vi "GCFS.vi"() -> ()   [LabVIEW 2024]
uses:
  Ice-Nucleation-Controller/src/LabVIEW/DataCluster_GCFS.ctl
  <vilib>/userDefined/High Color/IMAQdx.ctl
  <vilib>/vision/Image Controls.llb/IMAQ Image.ctl
  <vilib>/Platform/TimedLoop/XDataNode/timing_clust.ctl
  <vilib>/Platform/TimedLoop/XDataNode/nitl_modes.ctl
  <vilib>/Platform/TimedLoop/XDataNode/wakeup.ctl
  <vilib>/vision/driver/IMAQdx.llb/IMAQdx Buffer Number Mode.ctl
  <vilib>/addons/_JKI Toolkits/State Machine/_JKI_lib_State_Machine.llb/Select State(s)_err__jki_lib_state_machine.vi
  <extravilib>/ChannelInstances/Stream-c(t'IMAQ Image.ctl',str)/Read With Abort.vi
  <extravilib>/ChannelInstances/Tag-t'DataCluster_GCFS.ctl'/Read With Abort.vi
  <extravilib>/ChannelInstances/Stream-c(t'IMAQ Image.ctl',str)/Write With Abort.vi
  <extravilib>/ChannelInstances/Tag-t'DataCluster_GCFS.ctl'/Write With Abort.vi
  <extravilib>/ChannelInstances/Stream-c(t'IMAQ Image.ctl',str)/EndpointRead.vi
  <extravilib>/ChannelInstances/Stream-c(t'IMAQ Image.ctl',str)/Endpoint.vi
  <extravilib>/ChannelInstances/Stream-c(t'IMAQ Image.ctl',str)/Instantiate.vi
  <extravilib>/ChannelInstances/Tag-t'DataCluster_GCFS.ctl'/Instantiate.vi
  <extravilib>/ChannelInstances/Stream-c(t'IMAQ Image.ctl',str)/)Channel.vi
  <resource>/ChannelSupport/_ChannelSupport/WaitIfNeeded.vi
  <extravilib>/ChannelInstances/Tag-t'DataCluster_GCFS.ctl'/EndpointRead.vi
  <vilib>/addons/_JKI Toolkits/State Machine/_JKI_lib_State_Machine.llb/Periodic Trigger__ogtk__JKI-SM__jki_lib_state_machine.vi
  <extravilib>/ChannelInstances/Tag-t'DataCluster_GCFS.ctl'/Endpoint.vi
  <vilib>/platform/TimedLoop/XDataNode/XDataNode.xnode
  <vilib>/vision/driver/NI_Vision_Acquisition_Software.lvlib
  <extravilib>/ChannelInstances/Tag-t'DataCluster_GCFS.ctl'.lvlib
  <vilib>/vision/NI_Vision_Development_Module.lvlib
  <vilib>/Platform/TimedLoop/XDataNode/XDNodeRunTimeDep.lvlib
  <extravilib>/ChannelInstances/Stream-c(t'IMAQ Image.ctl',str).lvlib
panel:
  in  "Get Image":bool
  out "Frezz Image":T1(plugin-control)
  out "Droplet binary":T1(plugin-control)
  out "Droplet Position":T1(plugin-control)
  out "Grap Image":T1(plugin-control)
  in  "Active":bool
  in  "Sample name":string
  in  "Grap Position Image":bool
  out "Statusstring":string
  out "Particle Measurements (Pixels) (Particle Analysis 1)":dbl[][](array[numeric]) format="%.2f"
  out "Number of Particles":i32
  in  "Exit":bool
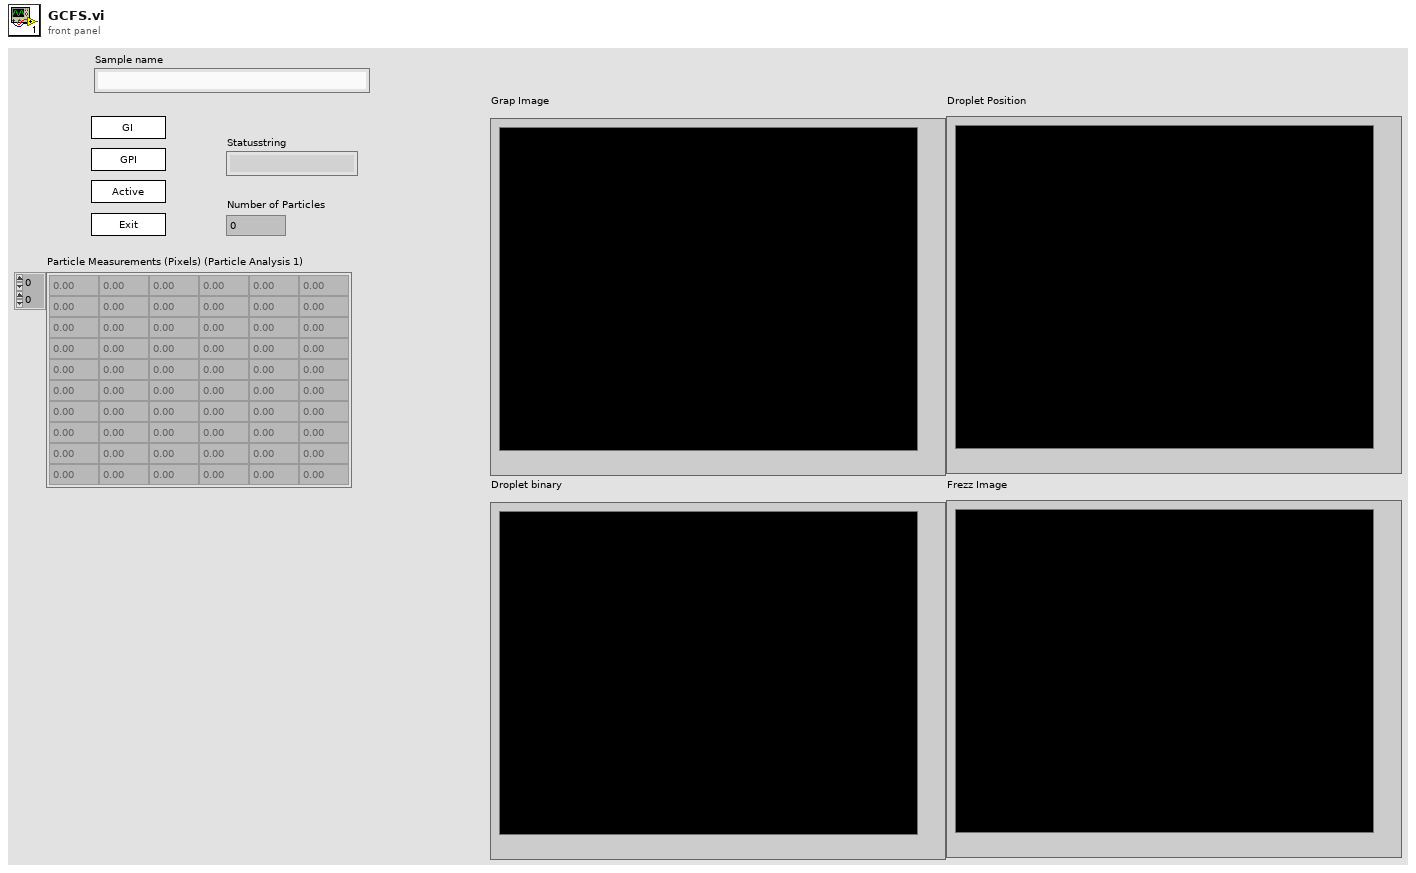
[diagram p1: front panel]
types:
  T1 = typedef "IMAQ Image.ctl" = refnum<image>
  T2 = typedef "DataCluster_GCFS.ctl" = cluster{"Core":cluster{"Current VI Reference":refnum<vi>, "Close Panel on Exit?":bool}, "Your Boolean data":bool, "Your string data":string, "Camera Cluster":cluster{"Session":T3, "Image":T1, "Position Image":T1, "PixelVal Image":T1, "Position Image Binary":T1}, "Data Cluster":cluster{"PosImg_Timestamp":string, "Particle Measurements (Pixels) (Particle Analysis 1)":dbl[][], "Images":cluster{"Position Image path":path, "Sample folder path":path}, "Number of droplets":i32, "Sample Name":string}, "Active":bool, "Ready":bool, "Exit":bool}
  T3 = typedef "IMAQdx.ctl" = refnum<k21>
  T4 = enum32{"Invalid", "Standard", "Closed", "Hidden", "Minimized", "Maximized"}
  T5 = enum32{"invalid app kind", "Development System", "Run Time System", "Student Edition", "Embedded LabVIEW", "Evaluation", "Custom"}
  T6 = cluster{"Current VI Reference":refnum<vi>, "Close Panel on Exit?":bool}
  T7 = typedef "Image Type" = u32
  T8 = cluster{"Type":u32, "Version":u32, "Flags":u32, "SerialNumberHigh":u32, "SerialNumberLow":u32, "BusType":u32, "InterfaceName":string, "VendorName":string, "ModelName":string, "CameraFileName":string, "CameraAttributeURL":string}[]
  T9 = typedef "Tag-t'DataCluster_GCFS.ctl'.lvlib/))Channel.ctl" = refnum<queue>
  T10 = cluster{"Image To Save":T1, "Snap timestamp":string}
  T11 = typedef "NI_Vision_Acquisition_Software.lvlib/IMAQdx Buffer Number Mode.ctl" = enum32{"Next", "Last", "Buffer Number", "Every", "Last New"}
  T12 = typedef "XDNodeRunTimeDep.lvlib/timing_clust.ctl" = cluster{"Expected End [f-1]":u64, "Actual End [f-1]":u64, "Finished Late? [f-1]":bool, "Expected End [i-1]":u64, "Actual End [i-1]":u64, "Finished Late? [i-1]":bool, "Expected Start [i]":u64, "Actual Start [i]":u64, "Expected Start [f]":u64, "Actual Start [f]":u64, "Source Name":string, "Structure Name":string, "Period":i64, "Deadline":i64, "Offset":i64, "Start":i64, "Priority":i32, "Timeout":i32, "Mode":T13, "Wakeup Reason":T14, "Error":errorcluster, "Source Type":string, "Secondary Source Type":string, "Global End Time":u64, "Global Start Time":u64, "Frame Duration":u64, "Iteration Duration":u64, "Assigned CPU":i32, "I/O Scan Engine Mode":u32}
  T13 = typedef "XDNodeRunTimeDep.lvlib/nitl_modes.ctl" = enum32{"No Change", "Process missed periods, maintain original phase", "Discard missed periods, maintain original phase", "Process missed periods, ignore original phase", "Discard missed periods, ignore original phase"}
  T14 = typedef "XDNodeRunTimeDep.lvlib/wakeup.ctl" = enum32{"Normal", "Aborted", "Asynchronous wakeup", "Timing source error", "Timed loop error", "Timeout"}
  T15 = typedef "Stream-c(t'IMAQ Image.ctl',str).lvlib/)Channel.ctl" = refnum<queue>
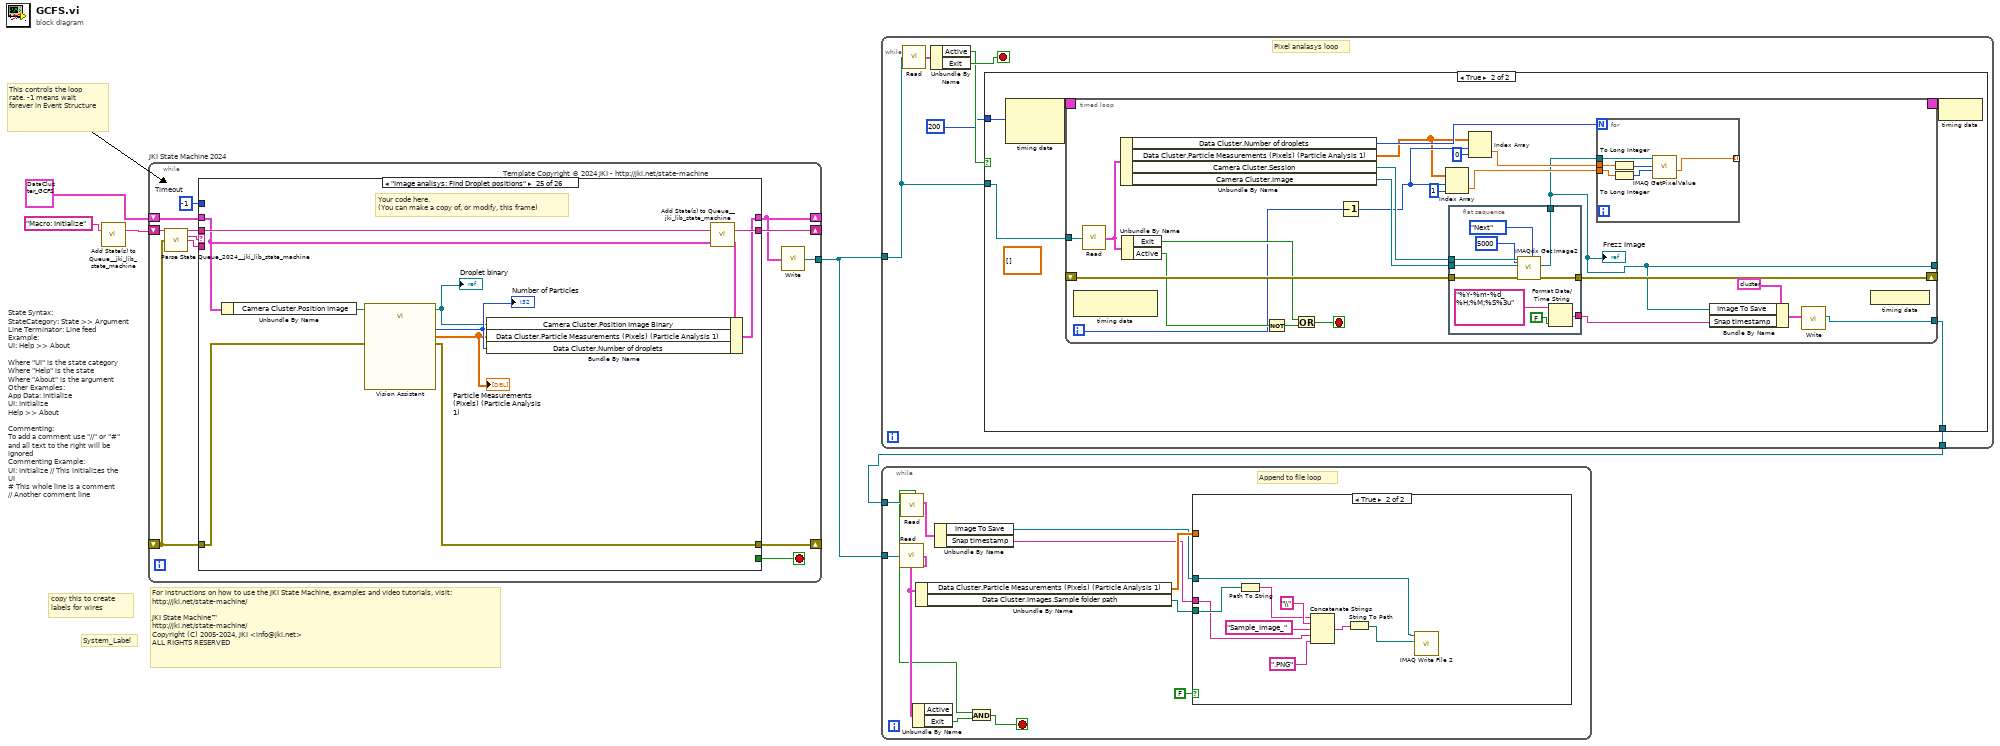
[diagram p0: block diagram]
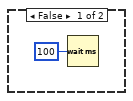
[diagram p2: hidden frame]
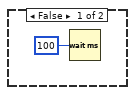
[diagram p3: hidden frame]
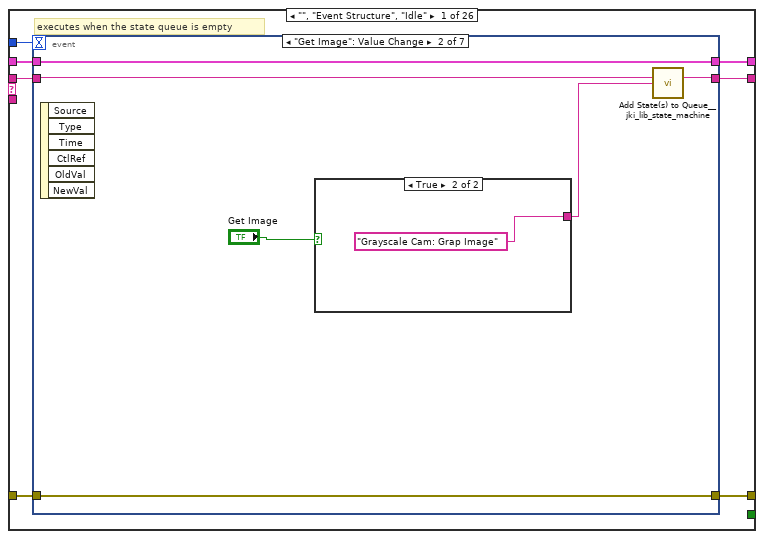
[diagram p4: hidden frame]
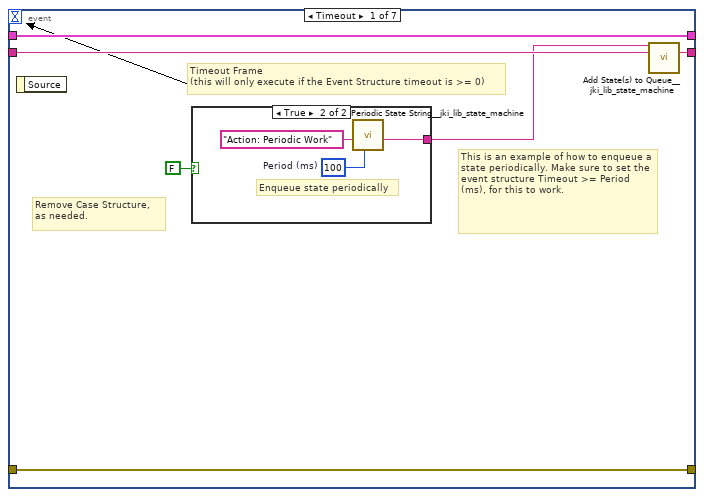
[diagram p5: hidden frame]
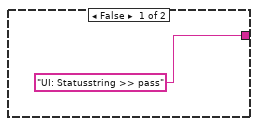
[diagram p7: hidden frame]
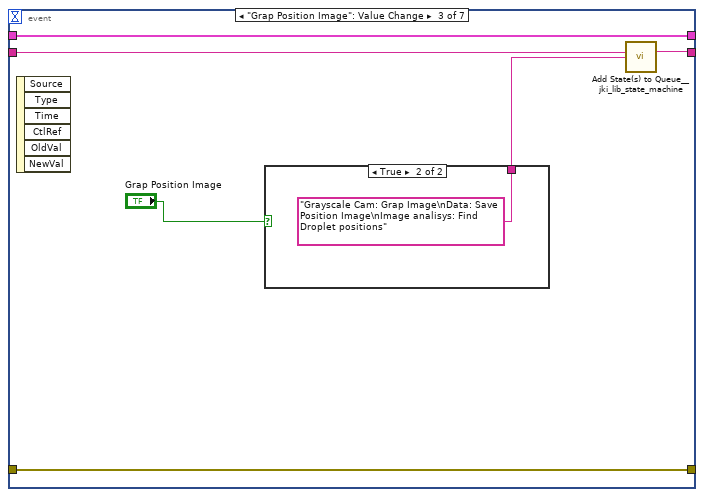
[diagram p8: hidden frame]
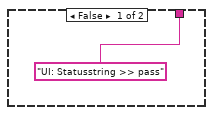
[diagram p9: hidden frame]
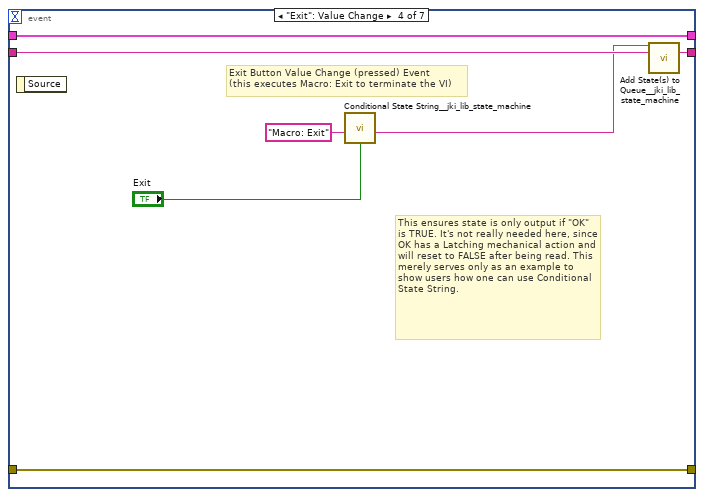
[diagram p10: hidden frame]
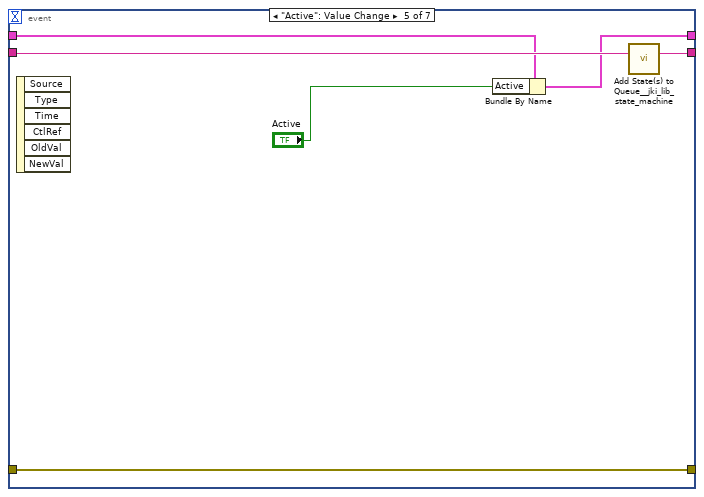
[diagram p11: hidden frame]
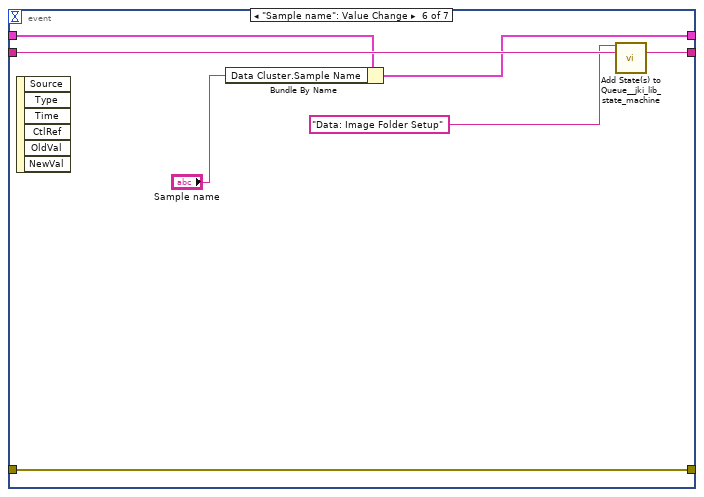
[diagram p12: hidden frame]
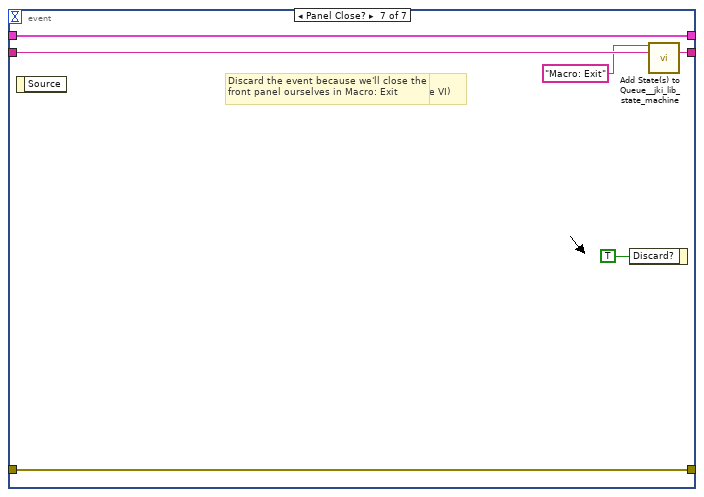
[diagram p13: hidden frame]
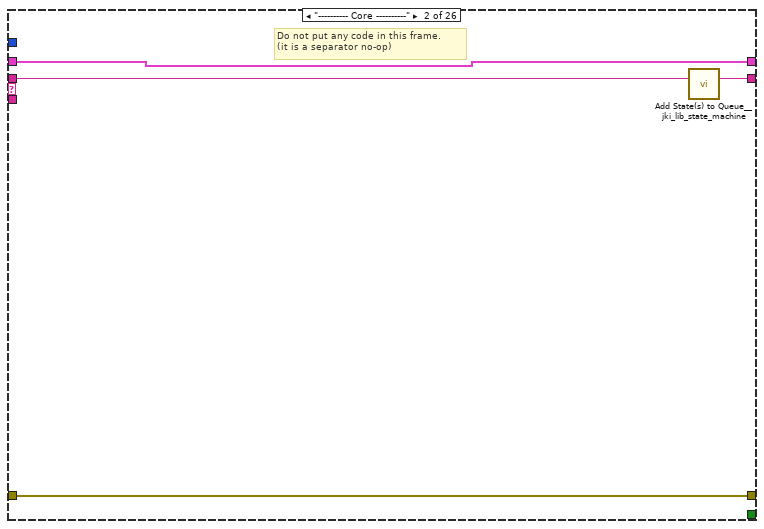
[diagram p14: hidden frame]
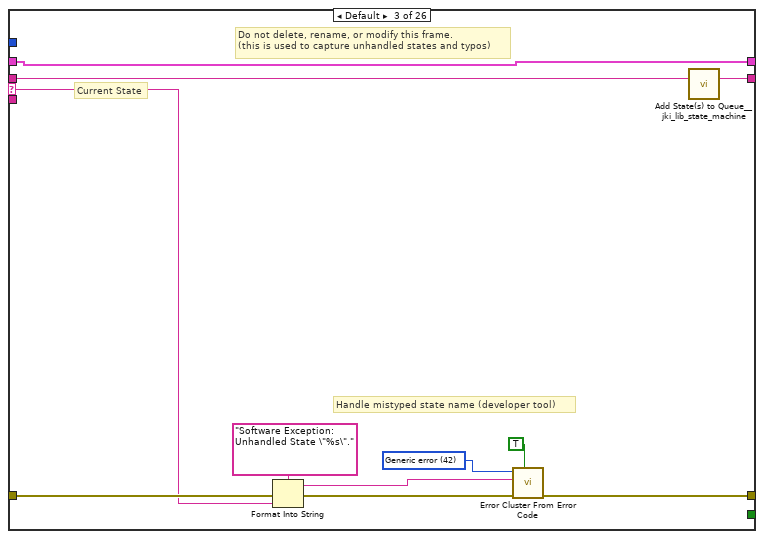
[diagram p15: hidden frame]
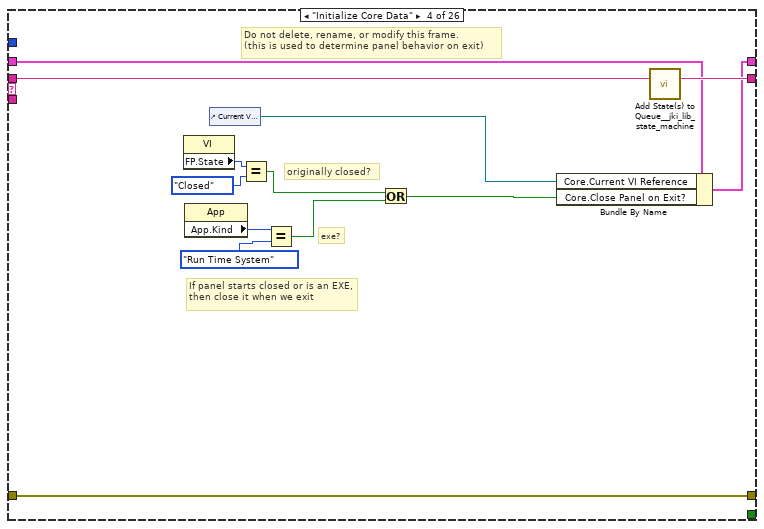
[diagram p16: hidden frame]
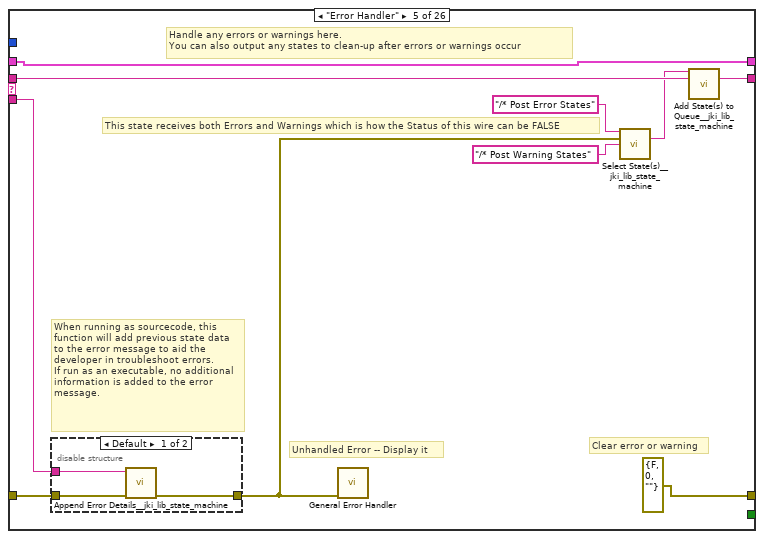
[diagram p17: hidden frame]
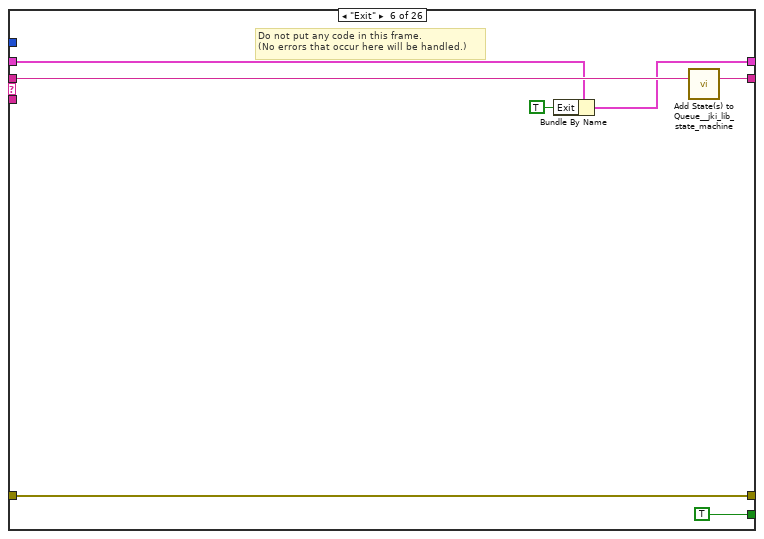
[diagram p19: hidden frame]
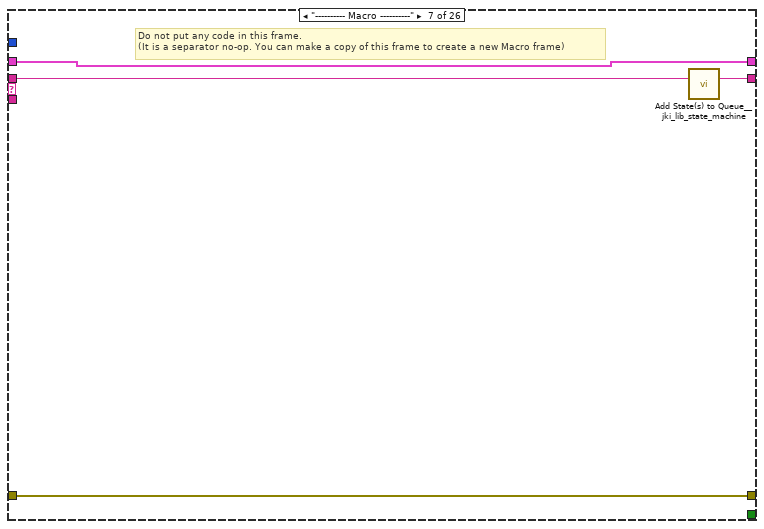
[diagram p20: hidden frame]
diagram:
  # "For instructions on how to use the JKI State Machine, examples and video tutorials, visit:\nhttp://jki.net/state-machine/\n\nJKI State Machine™\nhttp://jki.net/state-machine/\nCopyright (C) 2005-2024, JKI <info@jki.net>\nALL RIGHTS RESERVED"
  # "State Syntax:\nStateCategory: State >> Argument\nLine Terminator: Line feed\nExample:\nUI: Help >> About\n\nWhere \"UI\" is the state category\nWhere \"Help\" is the state\nWhere \"About\" is the argument\nOther Examples:\nApp Data: Initialize\nUI: Initialize\nHelp >> About\n\nCommenting:\nTo add a comment use \"//\" or \"#\" and all text to the right will be ignored\nCommenting Example:\nUI: Initialize // This initializes the UI\n# This whole line is a comment\n// Another comment line"
  # "copy this to create labels for wires"
  # "This controls the loop rate. -1 means wait forever in Event Structure"
  # "System_Label"
  n1 = call <vilib>:"Add State(s) to Queue__jki_lib_state_machine.vi"("State(s) in (\"\")"="Macro: Initialize") -> ("States Out"=w5:string)  [unwired: 14 in]
  n2 = while "JKI State Machine 2024" {
    shift-right: [w10] -> _
    shift-left: T2 {"Core"={"Current VI Reference"=refnum, "Close Panel on Exit?"=FALSE}, "Your Boolean data"=FALSE, "Your string data"="", "Camera Cluster"={"Session"="", "Image"=refnum, "Position Image"=refnum, "PixelVal Image"=refnum, "Position Image Binary"=refnum}, "Data Cluster"={"PosImg_Timestamp"="", "Particle Measurements (Pixels) (Particle Analysis 1)"=[], "Images"={"Position Image path"=path "", "Sample folder path"=path ""}, "Number of droplets"=0, "Sample Name"=""}, "Active"=FALSE, "Ready"=FALSE, "Exit"=FALSE} -> [w9]
    shift-right: [w13] -> _
    shift-left: _ -> [w7]
    shift-right: [w12] -> _
    shift-left: w5 -> [w14]
    tunnel: [w6] -> w2
    stop <- w11 stop-if-true
    w8 = -1  # Timeout
    # "Template Copyright © 2024 JKI - http://jki.net/state-machine"
    n3 = call <vilib>:"Parse State Queue_2024__jki_lib_state_machine.vi"("State Queue"=w14, "Error In (no error)"=w7) -> ("Remaining States"=w16:string, "Current State"=w17:string, "Arguments"=w15:string)  [unwired: 11 in]
    n4 = case shown="\"Image analisys: Find Droplet positions\"" w17 {
      selector: w17 -> [_ _ w80 _ _ _ _ _ _ _ _ _ _ _ _ _ _ _ _ _ _ _ _ _ _ _]
      tunnel: w16 -> [w24 w79 w84 w103 w113 w124 w128 w133 w142 w146 w157 w163 w180 w202 w206 w223 w227 w233 w244 w314 w318 w331 w356 w360 w370 w374]
      tunnel: w15 -> [_ _ _ _ w108 _ _ _ _ _ _ _ _ _ _ _ _ w228 w238 w310 _ _ _ _ _ _]
      tunnel: w9 -> [w22 w76 w82 w96 w110 w120 w125 w130 w140 w143 w153 w158 w166 w191 w203 w221 w225 w231 w240 w311 w315 w322 w347 w357 w365 w371]
      tunnel: [w21 w77 w86 w100 errorcluster {"status"=FALSE, "code"=0, "source"=""} ("error out") w122 w126 w131 w137 w144 w155 w159 w168 w192 w204 w214 w224 w229 w241 w312 w316 w319 w349 w358 w366 w372] -> w13
      tunnel: w7 -> [w18 w77 w85 w100 w109 w122 w126 w131 w137 w144 w155 w160 w170 w193 w204 w216 w224 w230 w242 w312 w316 w323 w351 w358 w367 w372]
      tunnel: [w23 w78 w83 w102 w112 w123 w127 w132 w141 w145 w156 w162 w179 w201 w205 w222 w226 w232 w243 w313 w317 w330 w355 w359 w369 w373] -> w12
      tunnel: [_ _ _ _ _ TRUE _ _ _ _ _ _ _ _ _ _ _ _ _ _ _ _ _ _ _ _] -> w11
      tunnel: [w20 w76 w82 w101 w110 w119 w125 w130 w140 w143 w152 w158 w165 w190 w203 w221 w225 w231 w240 w311 w315 w321 w348 w357 w364 w371] -> w10
      tunnel: w8 -> [w19 _ _ _ _ _ _ _ _ _ _ _ _ _ _ _ _ _ _ _ _ _ _ _ _ _]
      frame "", "Event Structure", "Idle" {
        # "executes when the state queue is empty"
        n5 = event shown="[1] \"Get Image\": Value Change" {
          selector: _ -> [_ _ _ _ _ _ _]
          dyn-events: _ -> [_ _ _ _ _ _ _]
          timeout: w19 -> [_ _ _ _ _ _ _]
          tunnel: w24 -> [w30 w36 w45 w56 w61 w68 w75]
          tunnel: [w29 w37 w46 w55 w62 w69 w74] -> w23
          tunnel: w22 -> [w27 w38 w47 w53 w60 w66 w72]
          tunnel: [w28 w39 w42 w54 w57 w63 w73] -> w21
          tunnel: w18 -> [w28 w39 w42 w54 w57 w63 w73]
          tunnel: [w27 w38 w47 w53 w59 w65 w72] -> w20
          event Timeout {
            # "Remove Case Structure, as needed."
            # "This is an example of how to enqueue a state periodically. Make sure to set the event structure Timeout >= Period (ms), for this to work."
            # "Timeout Frame\n(this will only execute if the Event Structure timeout is >= 0)"
            n6 = event-data() -> ()  [unwired: 1 in, 1 out]
            n7 = case shown="True" FALSE {
              tunnel: [_ w33] -> w26
              frame False {
              }
              frame True {
                w31 = u32 100  # Period (ms)
                # "Enqueue state periodically"
                n8 = call <vilib>:"Periodic State String__jki_lib_state_machine.vi"("Period (ms)"=w31, "State"="Action: Periodic Work") -> ("State Out"=w33:string)  [unwired: 9 in]
              }
            }
            n9 = call <vilib>:"Add State(s) to Queue__jki_lib_state_machine.vi"("State(s) in Front (\"\")"=w26, "State(s) in (\"\")"=w30) -> ("States Out"=w29:string)  [unwired: 13 in]
          }
          event "Get Image": Value Change {
            n10 = event-data() -> ()  [unwired: 1 in, 6 out]
            n11 = case shown="True" "Get Image" {
              tunnel: ["UI: Statusstring >> pass" "Grayscale Cam: Grap Image"] -> w35
              frame False {
              }
              frame True {
              }
            }
            n12 = call <vilib>:"Add State(s) to Queue__jki_lib_state_machine.vi"("State(s) in (\"\")"=w36, "State(s) at Back (\"\")"=w35) -> ("States Out"=w37:string)  [unwired: 13 in]
          }
          event "Grap Position Image": Value Change {
            n13 = event-data() -> ()  [unwired: 1 in, 6 out]
            n14 = case shown="True" "Grap Position Image" {
              tunnel: ["UI: Statusstring >> pass" "Grayscale Cam: Grap Image\nData: Save Position Image\nImage analisys: Find Droplet positions"] -> w43
              frame False {
              }
              frame True {
              }
            }
            n15 = call <vilib>:"Add State(s) to Queue__jki_lib_state_machine.vi"("State(s) in (\"\")"=w45, "State(s) at Back (\"\")"=w43) -> ("States Out"=w46:string)  [unwired: 13 in]
          }
          event "Exit": Value Change {
            # "This ensures state is only output if \"OK\" is TRUE. It's not really needed here, since OK has a Latching mechanical action and will reset to FALSE after being read. This merely serves only as an example to show users how one can use Conditional State String."
            # "Exit Button Value Change (pressed) Event\n(this executes Macro: Exit to terminate the VI)"
            n16 = event-data() -> ()  [unwired: 1 in, 1 out]
            n17 = call <vilib>:"Conditional State String__jki_lib_state_machine.vi"("Do State(s)?"="Exit", "State"="Macro: Exit") -> ("State Out"=w50:string)  [unwired: 7 in]
            n18 = call <vilib>:"Add State(s) to Queue__jki_lib_state_machine.vi"("State(s) in Front (\"\")"=w50, "State(s) in (\"\")"=w56) -> ("States Out"=w55:string)  [unwired: 13 in]
          }
          event "Active": Value Change {
            n19 = event-data() -> ()  [unwired: 1 in, 6 out]
            n20 = Bundle By Name(cluster=w60, "Active"="Active") -> (w59:T2)
            n21 = call <vilib>:"Add State(s) to Queue__jki_lib_state_machine.vi"("State(s) in (\"\")"=w61) -> ("States Out"=w62:string)  [unwired: 14 in]
          }
          event "Sample name": Value Change {
            n22 = event-data() -> ()  [unwired: 1 in, 6 out]
            n23 = Bundle By Name(cluster=w66, "Data Cluster.Sample Name"="Sample name") -> (w65:T2)
            n24 = call <vilib>:"Add State(s) to Queue__jki_lib_state_machine.vi"("State(s) in Front (\"\")"="Data: Image Folder Setup", "State(s) in (\"\")"=w68) -> ("States Out"=w69:string)  [unwired: 13 in]
          }
          event Panel Close? {
            # "Discard the event because we'll close the front panel ourselves in Macro: Exit"
            # "Close Panel button (pressed) Event\n(this executes Macro: Exit to terminate the VI)"
            n25 = event-data() -> ()  [unwired: 1 in, 1 out]
            n26 = event-data("Discard?"=TRUE) -> ()  [unwired: 1 in, 1 out]
            n27 = call <vilib>:"Add State(s) to Queue__jki_lib_state_machine.vi"("State(s) in Front (\"\")"="Macro: Exit", "State(s) in (\"\")"=w75) -> ("States Out"=w74:string)  [unwired: 13 in]
          }
        }
      }
      frame "---------- Core ----------" {
        # "Do not put any code in this frame.\n(it is a separator no-op)"
        n28 = call <vilib>:"Add State(s) to Queue__jki_lib_state_machine.vi"("State(s) in (\"\")"=w79) -> ("States Out"=w78:string)  [unwired: 14 in]
      }
      frame Default {
        w89 = 42 items=["No error", "Argument error", "Memory is full", "Out of zone", "End of file", "File already open", "Generic file I/O error", "File not found", "File permission error", "Disk is full", "Duplicate path", "Too many files open", "System feature not enabled", "Resource file not found", "Cannot add resource", "Resource not found", "Image not found", "Image memory error", "Pen does not exist", "Config type invalid", "Config token not found", "Config parse error", "Config memory error", "Bad external code format", "Bad external code offset", "External code not present", "Null window", "Destroy window error", "Null menu", "Print aborted", "Bad print record", "Print driver error", "Windows error during printing", "Memory error during printing", "Print dialog error", "Generic print error", "Invalid device refnum", "Device not found", "Device parameter error", "Device unit error", "Cannot open device", "Device call aborted", "Generic error", "Cancelled by user", "Object ID too low", "Object ID too high", "Object not in heap", "Unknown heap", "Unknown object (invalid DefProc)", "Unknown object (DefProc not in table)", "Message out of range", "Invalid (null) method", "Unknown message", "Manager call not supported", "Bad address", "Network operation in progress", "Network operation timed out", "Connection is busy", "Network attribute not supported", "Network error", "Address in use", "System out of memory", "Connection aborted", "Connection refused", "Not connected", "Already connected", "Connection closed", "Initialization error (interapplication manager)", "Bad occurrence", "Wait on unbound occurrence handler", "Occurrence queue overflow", "Datalog type conflict", "Unused", "Unrecognized type (interapplication manager)", "Memory corrupt", "Failed to make temporary DLL", "Old CIN version", "Drag socket not found", "Failed to load drop-object", "Failed to register OLE object", "Failed to release OLE object", "Format specifier type mismatch", "Unknown format specifier", "Too few format specifiers", "Too many format specifiers", "Scan failed", "Newer CIN version", "Error converting to variant", "Runtime menu error", "Password tampered", "Variant attribute not found", "Incompatible variant data type", "Event data is not available", "Event Store is not present", "Occurrence is not found", "Event Queue is not created", "Event info is not available", "Refnum passed is NULL", "Error retrieving Class GUID", "Error retrieving CoClass GUID", "Error retrieving TypeLib GUID.", "Bad built application magic bytes.", "Specific driver is different from the specific driver associated with the Logical Name.", "There is no session opened to the class driver.", "Max Error", "MAX - Error with config objects", "MAX - Error loading configuration", "MAX - Group not supported"]
        # "Current State"
        # "Do not delete, rename, or modify this frame.\n(this is used to capture unhandled states and typos)"
        # "Handle mistyped state name (developer tool)"
        n29 = Format Into String(format string="Software Exception: Unhandled State \"%s\"." ("message"), error in=w85, w80) -> (resulting string=w88:string, error out=w87:errorcluster)  [unwired: 1 in]
        n30 = call <vilib>:"Error Cluster From Error Code.vi"("show call chain? (False)"=TRUE, "error in (no error)"=w87, "error message (\"\")"=w88, "error code (0)"=w89) -> ("error out"=w86:errorcluster)  [unwired: 5 in]
        n31 = call <vilib>:"Add State(s) to Queue__jki_lib_state_machine.vi"("State(s) in (\"\")"=w84) -> ("States Out"=w83:string)  [unwired: 14 in]
      }
      frame "Initialize Core Data" {
        # "Do not delete, rename, or modify this frame.\n(this is used to determine panel behavior on exit)"
        # "originally closed?"
        # "exe?"
        # "If panel starts closed or is an EXE, then close it when we exit"
        n32 = property class="VI"() -> ("FP.State"=w93:T4)  [unwired: 2 in, 2 out]
        n33 = property class="App"() -> ("App.Kind"=w99:T5)  [unwired: 2 in, 2 out]
        n34 = control-ref of="Current VI Reference"() -> (w94:refnum<vi>)
        n35 = Equal?(x=w93, y=T4."Closed" ("Front Panel Window:State")) -> (x = y?=w91:bool)
        n36 = Equal?(x=w99, y=T5."Run Time System" ("Application:Kind")) -> (x = y?=w97:bool)
        n37 = Or(x=w91, y=w97) -> (x .or. y?=w95:bool)
        n38 = Bundle By Name(cluster=w96, "Core.Current VI Reference"=w94, "Core.Close Panel on Exit?"=w95) -> (w101:T2)
        n39 = call <vilib>:"Add State(s) to Queue__jki_lib_state_machine.vi"("State(s) in (\"\")"=w103) -> ("States Out"=w102:string)  [unwired: 14 in]
      }
      frame "Error Handler" {
        # "When running as sourcecode, this function will add previous state data to the error message to aid the developer in troubleshoot errors.\nIf run as an executable, no additional information is added to the error message."
        # "This state receives both Errors and Warnings which is how the Status of this wire can be FALSE"
        # "Unhandled Error -- Display it"
        # "Handle any errors or warnings here.\nYou can also output any states to clean-up after errors or warnings occur"
        # "Clear error or warning"
        n40 = disable-structure shown="Default" {
          disable-tunnel: w109 -> [w116 w117]
          disable-tunnel: w108 -> [w115 _]
          disable-tunnel: [w114 w117] -> w107
          frame condition #0 (active) {
            n41 = call <vilib>:"Append Error Details__jki_lib_state_machine.vi"("error in (no error)"=w116, "Previous State and Argument(s)"=w115) -> ("error out"=w114:errorcluster)  [unwired: 9 in]
          }
          frame condition #1 {
          }
        }
        n42 = call <vilib>:"General Error Handler.vi"("error in (no error)"=w107) -> ()  [unwired: 10 in, 5 out]
        n43 = call-poly <vilib>:"Select State(s)__jki_lib_state_machine.vi"("State(s) if True (\"\")"="/* Post Error States", "Select"=w107, "State(s) if False (\"\")"="/* Post Warning States") -> ("States Out"=w105:string)  [unwired: 12 in]
        n44 = call <vilib>:"Add State(s) to Queue__jki_lib_state_machine.vi"("State(s) in Front (\"\")"=w105, "State(s) in (\"\")"=w113) -> ("States Out"=w112:string)  [unwired: 13 in]
      }
      frame "Exit" {
        # "Do not put any code in this frame.\n(No errors that occur here will be handled.)"
        n45 = Bundle By Name(cluster=w120, "Exit"=TRUE) -> (w119:T2)
        n46 = call <vilib>:"Add State(s) to Queue__jki_lib_state_machine.vi"("State(s) in (\"\")"=w124) -> ("States Out"=w123:string)  [unwired: 14 in]
      }
      frame "---------- Macro ----------" {
        # "Do not put any code in this frame.\n(It is a separator no-op. You can make a copy of this frame to create a new Macro frame)"
        n47 = call <vilib>:"Add State(s) to Queue__jki_lib_state_machine.vi"("State(s) in (\"\")"=w128) -> ("States Out"=w127:string)  [unwired: 14 in]
      }
      frame "Macro: Initialize" {
        w129 = "Data: Initialize\nInitialize Core Data\nUI: Statusstring >> Initialysing\nUI: Front Panel State >> Open\nUI: Initialize\nData: Image Folder Setup\nGrayscale Cam: Initialize\nUI: Statusstring >> Initialysation done\n"  # Data: Initialize Initialize Core Data UI: Statusstring >> Initialysing UI: Front Panel State >> Open UI: Initialize Data: Image Folder Setup Grayscale Cam: Initialize UI: Statusstring >> Initialysation done
        # "Initialization Macro\n(This is called once, when the VI starts)"
        n48 = call <vilib>:"Add State(s) to Queue__jki_lib_state_machine.vi"("State(s) in Front (\"\")"=w129, "State(s) in (\"\")"=w133) -> ("States Out"=w132:string)  [unwired: 13 in]
      }
      frame "Macro: Exit" {
        # "Exit Macro\n(This is called once, when the VI exits)"
        n49 = Unbundle By Name(w140) -> ("Core.Close Panel on Exit?"=w135:bool)
        n50 = call <vilib>:"Conditional State String__jki_lib_state_machine.vi"("Do State(s)?"=w135, "State"="UI: Front Panel State >> Close") -> ("State Out"=w134:string)  [unwired: 7 in]
        n51 = call <vilib>:"Add State(s) to Queue__jki_lib_state_machine.vi"("State(s) in (\"\")"=w134, "State(s) at Back (\"\")"="UI: Uninitialize\nData: Cleanup\nExit") -> ("States Out"=w138:string)  [unwired: 13 in]
        n52 = call <vilib>:"Add State(s) to Queue__jki_lib_state_machine.vi"("State(s) in Front (\"\")"=w138, "State(s) in (\"\")"=w142) -> ("States Out"=w141:string)  [unwired: 13 in]
      }
      frame "---------- Data ----------" {
        # "Do not put any code in this frame.\n(It is a separator no-op. You can make a copy of this frame to create a new Data frame)"
        n53 = call <vilib>:"Add State(s) to Queue__jki_lib_state_machine.vi"("State(s) in (\"\")"=w146) -> ("States Out"=w145:string)  [unwired: 14 in]
      }
      frame "Data: Initialize" {
        w154 = T6 {"Current VI Reference"=refnum, "Close Panel on Exit?"=FALSE}  # Core
        # "do not delete - used by framework"
        # "Initialize the shift-register data, here.\n(data names are defined by what you wire into the bundle function)"
        n54 = local read "Sample name"() -> (w150:string)
        n55 = Equal?(x=w150, y="") -> (x = y?=w149:bool)
        n56 = call "Prompt User for Sample name"("Enable"=w149) -> ("Sample name"=w148:string)  [unwired: 16 in, 2 out]
        n57 = Select(t=w148, s=w149, f=w150) -> (s? t:f=w147:string)
        n58 = Bundle By Name(cluster=w153, "Core"=w154, "Data Cluster.Sample Name"=w147) -> (w152:T2)
        n59 = local write "Sample name"(w147) -> ()
        n60 = call <vilib>:"Add State(s) to Queue__jki_lib_state_machine.vi"("State(s) in (\"\")"=w157) -> ("States Out"=w156:string)  [unwired: 14 in]
      }
      frame "Data: Cleanup" {
        # "Cleanup any data and references, here.\n(this is called automatically, by the Macro: Exit)"
        n61 = Unbundle By Name(w158) -> ("Core.Current VI Reference"=w161:refnum<vi>)
        n62 = Close Reference(reference=w161, error in (no error)=w160) -> (error out=w159:errorcluster)
        n63 = call <vilib>:"Add State(s) to Queue__jki_lib_state_machine.vi"("State(s) in (\"\")"=w163) -> ("States Out"=w162:string)  [unwired: 14 in]
      }
      frame "Data: Image Folder Setup" {
        w173 = "\\" ("string")
        # "Do not put any code in this frame.\n(It is a separator no-op. You can make a copy of this frame to create a new Data frame)"
        n64 = Unbundle By Name(w166) -> ("Data Cluster.Sample Name"=w167:string)
        n65 = call <vilib>:"Application Directory.vi"() -> ("Application Directory"=w177:path)
        n66 = Path To String(path=w177) -> (string=w176:string)
        n67 = Concatenate Strings(w176, w173, "Flat Surface Images" ("string"), w173, w167) -> (w174:string)
        n68 = String To Path(string=w174) -> (path=w175:path)
        n69 = call <vilib>:"Check if File or Folder Exists.vi"("error in (no error)"=w170, "path"=w175) -> ("error out"=w169:errorcluster, "file or folder exists?"=w172:bool, "dup path"=w171:path)  [unwired: 7 in]
        n70 = case shown="True" w172 {
          tunnel: w171 -> [w182 w186]
          tunnel: w169 -> [w184 w185]
          tunnel: [w183 w185] -> w168
          tunnel: [w181 w186] -> w164
          frame False {
            n71 = Create Folder(path (use dialog)=w182, error in=w184) -> (created path=w181:path, error out=w183:errorcluster)  [unwired: 1 in, 1 out]
          }
          frame True {
          }
        }
        n72 = Bundle By Name(cluster=w166, "Data Cluster.Images.Sample folder path"=w164) -> (w165:T2)
        n73 = call <vilib>:"Add State(s) to Queue__jki_lib_state_machine.vi"("State(s) in (\"\")"=w180) -> ("States Out"=w179:string)  [unwired: 14 in]
      }
      frame "Data: Save Position Image" {
        # "Do not put any code in this frame.\n(It is a separator no-op. You can make a copy of this frame to create a new Data frame)"
        n74 = Unbundle By Name(w191) -> ("Camera Cluster.Image"=w196:T1, "Data Cluster.Images.Sample folder path"=w195:path, "Data Cluster.PosImg_Timestamp"=w194:string)
        n75 = Path To String(path=w195) -> (string=w197:string)
        n76 = Concatenate Strings(w197, "\\" ("string"), "Position_Image_" ("string"), w194, ".PNG" ("string")) -> (w200:string)
        n77 = String To Path(string=w200) -> (path=w189:path)
        n78 = call-poly "IMAQ Write File 2"("error in (no error)"=w193, "File Path"=w189, "Image"=w196) -> ("error out"=w192:errorcluster, "Image Out (duplicate)"=w187:T1)  [unwired: 7 in]
        "Droplet Position" <- w187
        n79 = Bundle By Name(cluster=w191, "Data Cluster.Images.Position Image path"=w189, "Camera Cluster.Position Image"=w187) -> (w190:T2)
        n80 = call <vilib>:"Add State(s) to Queue__jki_lib_state_machine.vi"("State(s) in (\"\")"=w202) -> ("States Out"=w201:string)  [unwired: 14 in]
      }
      frame "---------- UI ----------" {
        # "Do not put any code in this frame.\n(It is a separator no-op. You can make a copy of this frame to create a new UI frame)"
        n81 = call <vilib>:"Add State(s) to Queue__jki_lib_state_machine.vi"("State(s) in (\"\")"=w206) -> ("States Out"=w205:string)  [unwired: 14 in]
      }
      frame "UI: Initialize" {
        w210 = "\\" ("string")
        w218 = T7 6 items=["Grayscale (U8)", "Grayscale (I16)", "Grayscale (SGL)", "Complex (CSG)", "RGB (U32)", "HSL (U32)", "RGB (U64)", "Grayscale (U16)"] ("Image Type")
        w220 = T1 refnum ("Image")
        # "Initialize the User Interface, here.\n(this is called automatically, by the Macro: Initialize)"
        n82 = call <vilib>:"Application Directory.vi"() -> ("Application Directory"=w213:path)
        n83 = Path To String(path=w213) -> (string=w212:string)
        n84 = Concatenate Strings(w212, w210, "resources" ("string"), w210, "Logo_Full.png" ("string")) -> (w208:string)
        n85 = String To Path(string=w208) -> (path=w207:path)
        n86 = call "IMAQ Create"("Image Name"="Logo", "Image Type"=w218, "error in (no error)"=w216) -> ("New Image"=w217:T1, "error out"=w215:errorcluster)  [unwired: 2 in]
        n87 = call "IMAQ ReadFile 2"("File Path"=w207, "error in (no error)"=w215, "Image"=w217) -> ("error out"=w214:errorcluster)  [unwired: 4 in, 4 out]
        n88 = local write "Droplet binary"(w220) -> ()
        n89 = local write "Droplet Position"(w220) -> ()
        n90 = local write "Grap Image"(w220) -> ()
        n91 = local write "Frezz Image"(w220) -> ()
        n92 = call <vilib>:"Add State(s) to Queue__jki_lib_state_machine.vi"("State(s) in (\"\")"=w223) -> ("States Out"=w222:string)  [unwired: 14 in]
      }
      frame "UI: Uninitialize" {
        # "Cleanup the User Interface, here.\n(this is called automatically, by the Macro: Exit)"
        n93 = call <vilib>:"Add State(s) to Queue__jki_lib_state_machine.vi"("State(s) in (\"\")"=w227) -> ("States Out"=w226:string)  [unwired: 14 in]
      }
      frame "UI: Cursor Set" {
        # "Argument"
        # "Set and Unset Cursor Busy.\n(Usage: \"UI: Cursor Set >> Busy|Idle\")"
        n94 = case shown="\"Idle\", Default" w228 {
          tunnel: w230 -> [w235 w237]
          tunnel: [w234 w236] -> w229
          frame "Idle", Default {
            n95 = call <vilib>:"Unset Busy.vi"("error in (no error)"=w235) -> ("error out"=w234:errorcluster)  [unwired: 10 in]
          }
          frame "Busy" {
            n96 = call <vilib>:"Set Busy.vi"("error in (no error)"=w237) -> ("error out"=w236:errorcluster)  [unwired: 9 in, 1 out]
          }
        }
        n97 = call <vilib>:"Add State(s) to Queue__jki_lib_state_machine.vi"("State(s) in (\"\")"=w233) -> ("States Out"=w232:string)  [unwired: 14 in]
      }
      frame "UI: Front Panel State" {
        # "Argument"
        # "Set Front Panel Open or Closed\n(Usage: \"UI: Front Panel State >> Open|Close\")"
        n98 = Unbundle By Name(w240) -> ("Core.Current VI Reference"=w239:refnum<vi>)
        n99 = case shown="\"Open\", \"Standard\", Default" w238 {
          tunnel: w242 -> [w250 w265 w276 w289 w302]
          tunnel: [w252 w266 w278 w291 w304] -> w241
          tunnel: w239 -> [w251 w263 w277 w290 w303]
          frame "Open", "Standard", Default {
            w245 = T4."Standard" ("State")
            n100 = property class="VI"(reference=w251, error in=w250) -> (reference out=w248:refnum<vi>, error out=w249:errorcluster, "FP.State"=w247:T4)
            n101 = Not Equal?(x=w247, y=w245) -> (x != y?=w246:bool)
            n102 = case shown="False" w246 {
              tunnel: [w256 w258] -> w252
              tunnel: w249 -> [w255 w258]
              tunnel: w248 -> [w254 _]
              tunnel: w245 -> [w253 _]
              frame True {
                n103 = invoke class="VI" method="FP.Open"(reference=w254, error in=w255, "Activate"=TRUE, "State"=w253) -> (error out=w256:errorcluster)  [unwired: 1 in, 4 out]
              }
              frame False {
              }
            }
          }
          frame "Close", "Closed" {
            n104 = property class="VI"(reference=w263, error in=w265) -> (reference out=w262:refnum<vi>, error out=w264:errorcluster, "FP.State"=w260:T4)
            n105 = Not Equal?(x=w260, y=T4."Closed" ("Front Panel Window:State")) -> (x != y?=w259:bool)
            n106 = case shown="True" w259 {
              tunnel: [w267 w270] -> w266
              tunnel: w264 -> [w267 w269]
              tunnel: w262 -> [_ w268]
              frame False {
              }
              frame True {
                n107 = invoke class="VI" method="FP.Close"(reference=w268, error in=w269) -> (error out=w270:errorcluster)  [unwired: 1 in, 2 out]
              }
            }
          }
          frame "Hidden", "Hide" {
            w271 = T4."Hidden" ("State")
            n108 = property class="VI"(reference=w277, error in=w276) -> (reference out=w274:refnum<vi>, error out=w275:errorcluster, "FP.State"=w273:T4)
            n109 = Not Equal?(x=w273, y=w271) -> (x != y?=w272:bool)
            n110 = case shown="True" w272 {
              tunnel: [w282 w283] -> w278
              tunnel: w275 -> [w281 w283]
              tunnel: w274 -> [w280 _]
              tunnel: w271 -> [w279 _]
              frame True {
                n111 = invoke class="VI" method="FP.Open"(reference=w280, error in=w281, "State"=w279) -> (error out=w282:errorcluster)  [unwired: 2 in, 4 out]
              }
              frame False {
              }
            }
          }
          frame "Minimize", "Minimized" {
            w284 = T4."Minimized" ("State")
            n112 = property class="VI"(reference=w290, error in=w289) -> (reference out=w287:refnum<vi>, error out=w288:errorcluster, "FP.State"=w286:T4)
            n113 = Not Equal?(x=w286, y=w284) -> (x != y?=w285:bool)
            n114 = case shown="True" w285 {
              tunnel: [w295 w296] -> w291
              tunnel: w288 -> [w294 w296]
              tunnel: w287 -> [w293 _]
              tunnel: w284 -> [w292 _]
              frame True {
                n115 = invoke class="VI" method="FP.Open"(reference=w293, error in=w294, "State"=w292) -> (error out=w295:errorcluster)  [unwired: 2 in, 4 out]
              }
              frame False {
              }
            }
          }
          frame "Maximize", "Maximized" {
            w297 = T4."Maximized" ("State")
            n116 = property class="VI"(reference=w303, error in=w302) -> (reference out=w300:refnum<vi>, error out=w301:errorcluster, "FP.State"=w299:T4)
            n117 = Not Equal?(x=w299, y=w297) -> (x != y?=w298:bool)
            n118 = case shown="True" w298 {
              tunnel: [w308 w309] -> w304
              tunnel: w301 -> [w307 w309]
              tunnel: w300 -> [w306 _]
              tunnel: w297 -> [w305 _]
              frame True {
                n119 = invoke class="VI" method="FP.Open"(reference=w306, error in=w307, "State"=w305) -> (error out=w308:errorcluster)  [unwired: 2 in, 4 out]
              }
              frame False {
              }
            }
          }
        }
        n120 = call <vilib>:"Add State(s) to Queue__jki_lib_state_machine.vi"("State(s) in (\"\")"=w244) -> ("States Out"=w243:string)  [unwired: 14 in]
      }
      frame "UI: Statusstring" {
        # "Do not put any code in this frame.\n(It is a separator no-op. You can make a copy of this frame to create a new UI frame)"
        n121 = call <vilib>:"Add State(s) to Queue__jki_lib_state_machine.vi"("State(s) in (\"\")"=w314) -> ("States Out"=w313:string)  [unwired: 14 in]
        "Statusstring" <- w310
      }
      frame "---------- Grayscale Cam ----------" {
        # "Template Separator\n(You can make a copy of, or modify, this frame)"
        n122 = call <vilib>:"Add State(s) to Queue__jki_lib_state_machine.vi"("State(s) in (\"\")"=w318) -> ("States Out"=w317:string)  [unwired: 14 in]
      }
      frame "Grayscale Cam: Initialize" {
        # "Template Separator\n(You can make a copy of, or modify, this frame)"
        n123 = call <vilib>:"IMAQdx Enumerate Cameras.vi"("error in"=w323) -> ("error out"=w324:errorcluster, "Camera Information Array"=w328:T8)  [unwired: 9 in]
        n124 = Array Size(array=w328) -> (size(s)=w329:i32)
        n125 = for {
          N: w329 -> [_]
          tunnel: w328 -> [w339] mode=indexing
          shift-right: [w337] -> w327
          shift-left: _ -> [w332]
          n126 = Unbundle By Name(w339) -> ("InterfaceName"=w338:string, "VendorName"=w336:string)
          n127 = Match True/False String(2:"" ("false string"), 3:"JAI" ("true string"), 4:w336) -> (0:w333:bool)  [unwired: 1 out]
          n128 = Select(t=w338, s=w333, f=w332) -> (s? t:f=w337:string)
        }
        n129 = call <vilib>:"IMAQdx Open Camera.vi"("error in"=w324, "Session In"=w327) -> ("error out"=w326:errorcluster, "Session Out"=w325:T3)  [unwired: 8 in]
        n130 = call <vilib>:"IMAQdx Configure Grab.vi"("error in"=w326, "Session In"=w325) -> ("error out"=w319:errorcluster, "Session Out"=w320:T3)  [unwired: 8 in]
        n131 = Bundle By Name(cluster=w322, "Camera Cluster.Session"=w320) -> (w321:T2)
        n132 = call <vilib>:"Add State(s) to Queue__jki_lib_state_machine.vi"("State(s) in (\"\")"=w331) -> ("States Out"=w330:string)  [unwired: 14 in]
      }
      frame "Grayscale Cam: Grap Image" {
        w353 = T7 0 items=["Grayscale (U8)", "Grayscale (I16)", "Grayscale (SGL)", "Complex (CSG)", "RGB (U32)", "HSL (U32)", "RGB (U64)", "Grayscale (U16)"] ("Image Type")
        # "Template Separator\n(You can make a copy of, or modify, this frame)"
        n133 = Unbundle By Name(w347) -> ("Camera Cluster.Session"=w346:T3)
        n134 = call "IMAQ Create"("Image Name"="Image", "Image Type"=w353, "error in (no error)"=w351) -> ("New Image"=w352:T1, "error out"=w350:errorcluster)  [unwired: 2 in]
        n135 = Format Date/Time String(time format string (%c)="%Y-%m-%d_%H;%M;%S%3u", UTC format=FALSE) -> (date/time string=w341:string)  [unwired: 1 in]
        n136 = call <vilib>:"IMAQdx Grab2.vi"("Timeout (ms)"=5000, "error in"=w350, "Image In"=w352, "Session In"=w346) -> ("error out"=w349:errorcluster, "Image Out"=w340:T1, "Session Out"=w345:T3)  [unwired: 4 in, 1 out]
        "Grap Image" <- w340
        n137 = Bundle By Name(cluster=w347, "Camera Cluster.Session"=w345, "Camera Cluster.Image"=w340, "Data Cluster.PosImg_Timestamp"=w341) -> (w348:T2)
        n138 = call <vilib>:"Add State(s) to Queue__jki_lib_state_machine.vi"("State(s) in (\"\")"=w356) -> ("States Out"=w355:string)  [unwired: 14 in]
      }
      frame "---------- Image analisys ----------" {
        # "Template Separator\n(You can make a copy of, or modify, this frame)"
        n139 = call <vilib>:"Add State(s) to Queue__jki_lib_state_machine.vi"("State(s) in (\"\")"=w360) -> ("States Out"=w359:string)  [unwired: 14 in]
      }
      frame "Image analisys: Find Droplet positions" {
        # "Your code here.\n(You can make a copy of, or modify, this frame)"
        n140 = Unbundle By Name(w365) -> ("Camera Cluster.Position Image"=w368:T1)
        n141 = call "Vision Assistant"("Image In"=w368, "error in"=w367) -> ("Image Out"=w361:T1, "Number of Particles (Particle Analysis 1)"=w363:i32, "Particle Measurements (Pixels) (Particle Analysis 1)"=w362:dbl[][], "error out"=w366:errorcluster)  [unwired: 20 in, 2 out]
        "Number of Particles" <- w363
        "Particle Measurements (Pixels) (Particle Analysis 1)" <- w362
        "Droplet binary" <- w361
        n142 = Bundle By Name(cluster=w365, "Camera Cluster.Position Image Binary"=w361, "Data Cluster.Particle Measurements (Pixels) (Particle Analysis 1)"=w362, "Data Cluster.Number of droplets"=w363) -> (w364:T2)
        n143 = call <vilib>:"Add State(s) to Queue__jki_lib_state_machine.vi"("State(s) in (\"\")"=w370) -> ("States Out"=w369:string)  [unwired: 14 in]
      }
      frame "Image analisys: 2" {
        # "Your code here.\n(You can make a copy of, or modify, this frame)"
        n144 = call <vilib>:"Add State(s) to Queue__jki_lib_state_machine.vi"("State(s) in (\"\")"=w374) -> ("States Out"=w373:string)  [unwired: 14 in]
      }
    }
    n145 = call <extravilib>:"Write.vi"("element"=w10) -> ("channel"=w6:T9)  [unwired: 1 out]
  }
  n146 = while {
    tunnel: w2 -> [w380]
    tunnel: [w375] -> w1
    stop <- w378 stop-if-true
    # "Pixel analasys loop"
    n147 = call <extravilib>:"Read.vi"("channel"=w380) -> ("element"=w379:T2)  [unwired: 1 in, 1 out]
    n148 = Unbundle By Name(w379) -> ("Active"=w377:bool, "Exit"=w378:bool)
    n149 = case shown="True" w377 {
      tunnel: w380 -> [_ w386]
      tunnel: i64 200 ("Period") -> [_ w383]
      tunnel: [_ w382] -> w375
      frame False {
        n150 = Wait (ms)(milliseconds to wait=u32 100) -> ()  [unwired: 1 out]
      }
      frame True {
        (unwired) sgl[][] []
        n151 = node-c288(w383) -> (w385:T12)  [unwired: 1 in]
        n152 = timed-loop {
          tunnel: w386 -> [w409]
          shift-right: [w405] -> _
          shift-left: _ -> [w406]
          timing: w385 -> [_]
          timing-out: [_] -> w384
          tunnel: [w389] -> _
          tunnel: [w387] -> w382
          i -> [w397]
          stop <- w392 stop-if-true
          n153 = node-c288() -> ()  [unwired: 1 in, 1 out]
          n154 = call <extravilib>:"Read.vi"("channel"=w409) -> ("element"=w402:T2)  [unwired: 1 in, 1 out]
          n155 = Unbundle By Name(w402) -> ("Data Cluster.Number of droplets"=w404:i32, "Data Cluster.Particle Measurements (Pixels) (Particle Analysis 1)"=w395:dbl[][], "Camera Cluster.Session"=w408:T3, "Camera Cluster.Image"=w407:T1)
          n156 = Unbundle By Name(w402) -> ("Exit"=w400:bool, "Active"=w401:bool)
          n157 = Not(x=w401) -> (.not. x?=w403:bool)
          n158 = Or(x=w400, y=w403) -> (x .or. y?=w392:bool)
          n159 = Decrement(x=w397) -> (x-1=w396:i32)
          n160 = Index Array(array=w395, index (row)=w396, index (col)=1) -> (element=w394:dbl)
          n161 = flat-sequence {
            tunnel: w408 -> [w424]
            tunnel: w407 -> [w423]
            tunnel: w406 -> [w421]
            tunnel: [w420] -> w405
            tunnel: [w419] -> w389
            tunnel: [w416] -> w390
            frame #0 {
              n162 = call <vilib>:"IMAQdx Get Image2.vi"("Timeout (ms)"=5000, "Buffer Number Mode (Next)"=IMAQdx_Buffer_Number_Mode."Next", "error in"=w421, "Image In"=w423, "Session In"=w424) -> ("error out"=w420:errorcluster, "Image Out"=w419:T1)  [unwired: 3 in, 2 out]
              n163 = Format Date/Time String(time format string (%c)="%Y-%m-%d_%H;%M;%S%3u", UTC format=FALSE) -> (date/time string=w416:string)  [unwired: 1 in]
            }
          }
          n164 = Index Array(array=w395, index (row)=w396, index (col)=0 ("disabled index (col)")) -> (element=w393:dbl)
          n165 = for {
            N: w404 -> [_]
            tunnel: w389 -> [w415]
            tunnel: w394 -> [w412]
            tunnel: w393 -> [w414]
            tunnel: [w410] -> _ mode=indexing
            n166 = To Long Integer(number=w414) -> (32bit integer=w413:i32)
            n167 = To Long Integer(number=w412) -> (32bit integer=w411:i32)
            n168 = call "IMAQ GetPixelValue"("Image"=w415, "X Coordinate"=w413, "Y Coordinate"=w411) -> ("Pixel Value (Float)"=w410:sgl)  [unwired: 3 in, 4 out]
          }
          n169 = Bundle By Name(cluster=T10 {"Image To Save"=refnum, "Snap timestamp"=""}, "Image To Save"=w389, "Snap timestamp"=w390) -> (w388:T10)
          n170 = call <extravilib>:"Write.vi"("element"=w388) -> ("channel"=w387:T15)  [unwired: 8 in, 2 out]
          n171 = node-c288() -> ()  [unwired: 1 out]
          "Frezz Image" <- w389
        }
        n172 = node-c288(w384) -> ()
      }
    }
  }
  n173 = while {
    tunnel: w2 -> [w443]
    tunnel: w1 -> [w436]
    stop <- w433 stop-if-true
    # "Append to file loop"
    n174 = call <extravilib>:"Read.vi"("channel"=w443) -> ("element"=w442:T2)  [unwired: 1 in, 1 out]
    n175 = call <extravilib>:"Read.vi"("channel"=w436) -> ("element"=w435:T10, "timed out?"=w432:bool)  [unwired: 6 in, 3 out]
    n176 = Unbundle By Name(w442) -> ("Exit"=w434:bool)  [unwired: 1 out]
    n177 = Unbundle By Name(w442) -> ("Data Cluster.Particle Measurements (Pixels) (Particle Analysis 1)"=w441:dbl[][], "Data Cluster.Images.Sample folder path"=w438:path)
    n178 = Unbundle By Name(w435) -> ("Image To Save"=w440:T1, "Snap timestamp"=w439:string)
    n179 = And(x=w432, y=w434) -> (x .and. y?=w433:bool)
    n180 = case shown="True" FALSE {
      tunnel: w441 -> [_ _]
      tunnel: w440 -> [_ w446]
      tunnel: w439 -> [_ w447]
      tunnel: w438 -> [_ w448]
      frame False {
        n181 = Wait (ms)(milliseconds to wait=u32 100) -> ()  [unwired: 1 out]
      }
      frame True {
        n182 = Path To String(path=w448) -> (string=w450:string)
        n183 = Concatenate Strings(w450, "\\" ("string"), "Sample_Image_" ("string"), w447, ".PNG" ("string")) -> (w453:string)
        n184 = String To Path(string=w453) -> (path=w449:path)
        n185 = call-poly "IMAQ Write File 2"("File Path"=w449, "Image"=w446) -> ()  [unwired: 8 in, 2 out]
      }
    }
  }
